vi "number from rotated int string (SubVI).vi"(5 "String":string="00000190") -> (0 "int number":i32, 1 "Rotated int String":string, 2 "rotated int number":i32)   [LabVIEW 2017, in "LV_Unicorn.lvlib"]
uses:
  LV_Unicorn.lvlib
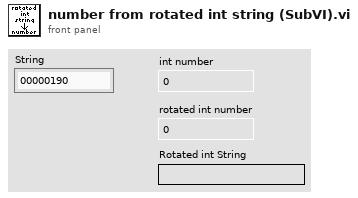
[diagram p1: front panel]
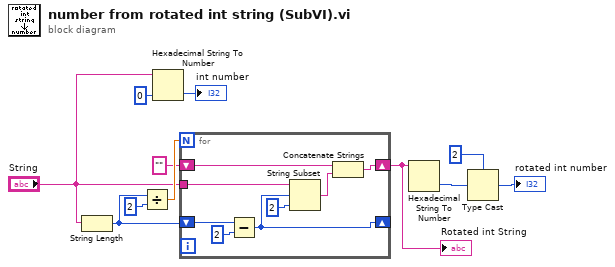
[diagram p0: block diagram]
diagram:
  n1 = String Length(string="String") -> (length=w8:i32)
  n2 = Divide(x=w8, y=2) -> (x/y=w10:dbl)
  n3 = Hexadecimal String To Number(string="String", default (0uL)=0 ("default (0 U32)")) -> (number=→"int number":i32)  [unwired: 1 in, 1 out]
  n4 = for {
    N: w10 -> [_]
    tunnel: "String" -> [w19]
    shift-right: [w12] -> _
    shift-left: w8 -> [w18]
    shift-right: [w13] -> w6
    shift-left: "" -> [w15]
    n5 = Subtract(x=w18, y=2) -> (x-y=w12:i32)
    n6 = String Subset(string=w19, offset (0)=w12, length (rest)=2 ("length (rest)")) -> (substring=w14:string)
    n7 = Concatenate Strings(w15, w14) -> (w13:string)
  }
  "Rotated int String" <- w6
  n8 = Hexadecimal String To Number(string=w6) -> (number=w4:u32)  [unwired: 2 in, 1 out]
  n9 = Type Cast(type=2, x=w4) -> (*(type *) &x=→"rotated int number":i32)
